vi "WaveForm.vi"(0 "time(ms)":dbl, 1 "amplitude":dbl, 2 "offset":dbl, 3 "frequency":dbl, 4 "waveform":enum16{"sin", "square"}(ring)) -> (5 "wave":dbl)   [LabVIEW 2020]
panel:
  out "oldwave":dbl
  out "oldsin":dbl
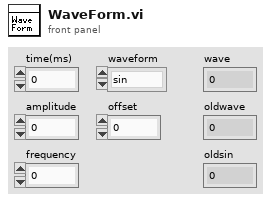
[diagram p1: front panel]
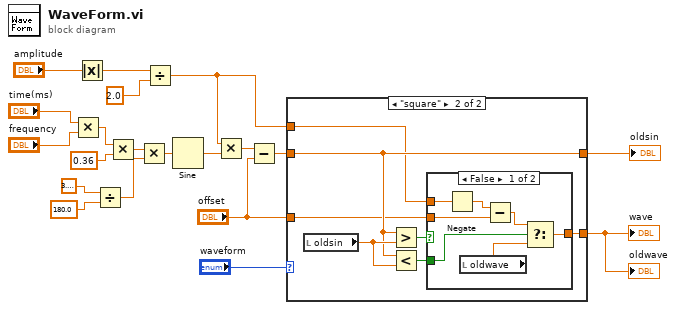
[diagram p0: block diagram]
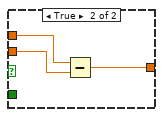
[diagram p3: hidden frame]
diagram:
  n1 = Multiply(x="time(ms)", y="frequency") -> (x*y=w2:dbl)
  n2 = Absolute Value(x="amplitude") -> (abs(x)=w9:dbl)
  n3 = Divide(x=3.141592653589793, y=180.0) -> (x/y=w5:dbl)
  n4 = Multiply(x=w2, y=0.36) -> (x*y=w1:dbl)
  n5 = Multiply(x=w1, y=w5) -> (x*y=w4:dbl)
  n6 = Divide(x=w9, y=2.0) -> (x/y=w12:dbl)
  n7 = Sine(x=w4) -> (sin(x)=w17:dbl)
  n8 = Multiply(x=w12, y=w17) -> (x*y=w13:dbl)
  n9 = Subtract(x=w13, y="offset") -> (x-y=w14:dbl)
  n10 = case shown="\"square\"" "waveform" {
    tunnel: [w21 w22] -> w8
    tunnel: w14 -> [w21 w25]
    tunnel: w12 -> [_ w24]
    tunnel: "offset" -> [_ w23]
    tunnel: [w21 w25] -> w10
    frame "sin", Default {
    }
    frame "square" {
      n11 = local read "oldsin"() -> (w26:dbl)
      n12 = Greater?(x=w25, y=w26) -> (0:w28:bool)
      n13 = Less?(x=w25, y=w26) -> (x < y?=w27:bool)
      n14 = case shown="FALSE" w28 {
        tunnel: [w35 w36] -> w22
        tunnel: w27 -> [w29 _]
        tunnel: w24 -> [w34 w38]
        tunnel: w23 -> [w32 w37]
        frame False {
          n15 = Negate(x=w34) -> (-x=w33:dbl)
          n16 = local read "oldwave"() -> (w30:dbl)
          n17 = Subtract(x=w33, y=w32) -> (x-y=w31:dbl)
          n18 = Select(t=w31, s=w29, f=w30) -> (s? t:f=w35:dbl)
        }
        frame True {
          n19 = Subtract(x=w38, y=w37) -> (x-y=w36:dbl)
        }
      }
    }
  }
  "wave" <- w8
  "oldsin" <- w10
  "oldwave" <- w8
